vi "Meas Result Get Readings.vi"(5 "table ref":refnum<vi>, 6 "equ cct":T1, 7 "formats":T3={"mjr fmt"=enum."%_5p", "mnr fmt"=enum."%_5p", "iref fmt"=enum."%_5p", "udut fmt"=enum."%_5p", "udvm fmt"=enum."%_5p"}, 8 "error in (no error)":errorcluster, 9 "ring spot":refnum<vi>, 10 "ring phase":refnum<vi>, 11 "result":T6) -> (0 "error out":errorcluster, 1 "sweep spot index":u16, 2 "phase index":u16, 3 "readings":T4, 4 "quantities":T5)   [LabVIEW 2020]
doc: "Gets readings for selected sweep spot."
uses:
  Meas Results.ctl
  bridge/Bridge Frequency Readings Data.ctl
  drivers/TWM client/Meas Proc QWTB Spectrum Data.ctl
  drivers/TWM client/TWM Phase Info.ctl
  Meas Quantity Names.ctl
  Meas Result Formats.ctl
  Meas Result Major Format.ctl
  Impedance Equivalent Circuit.ctl
panel:
  in  "fmt":T2=enum."%_5p" caption="format"
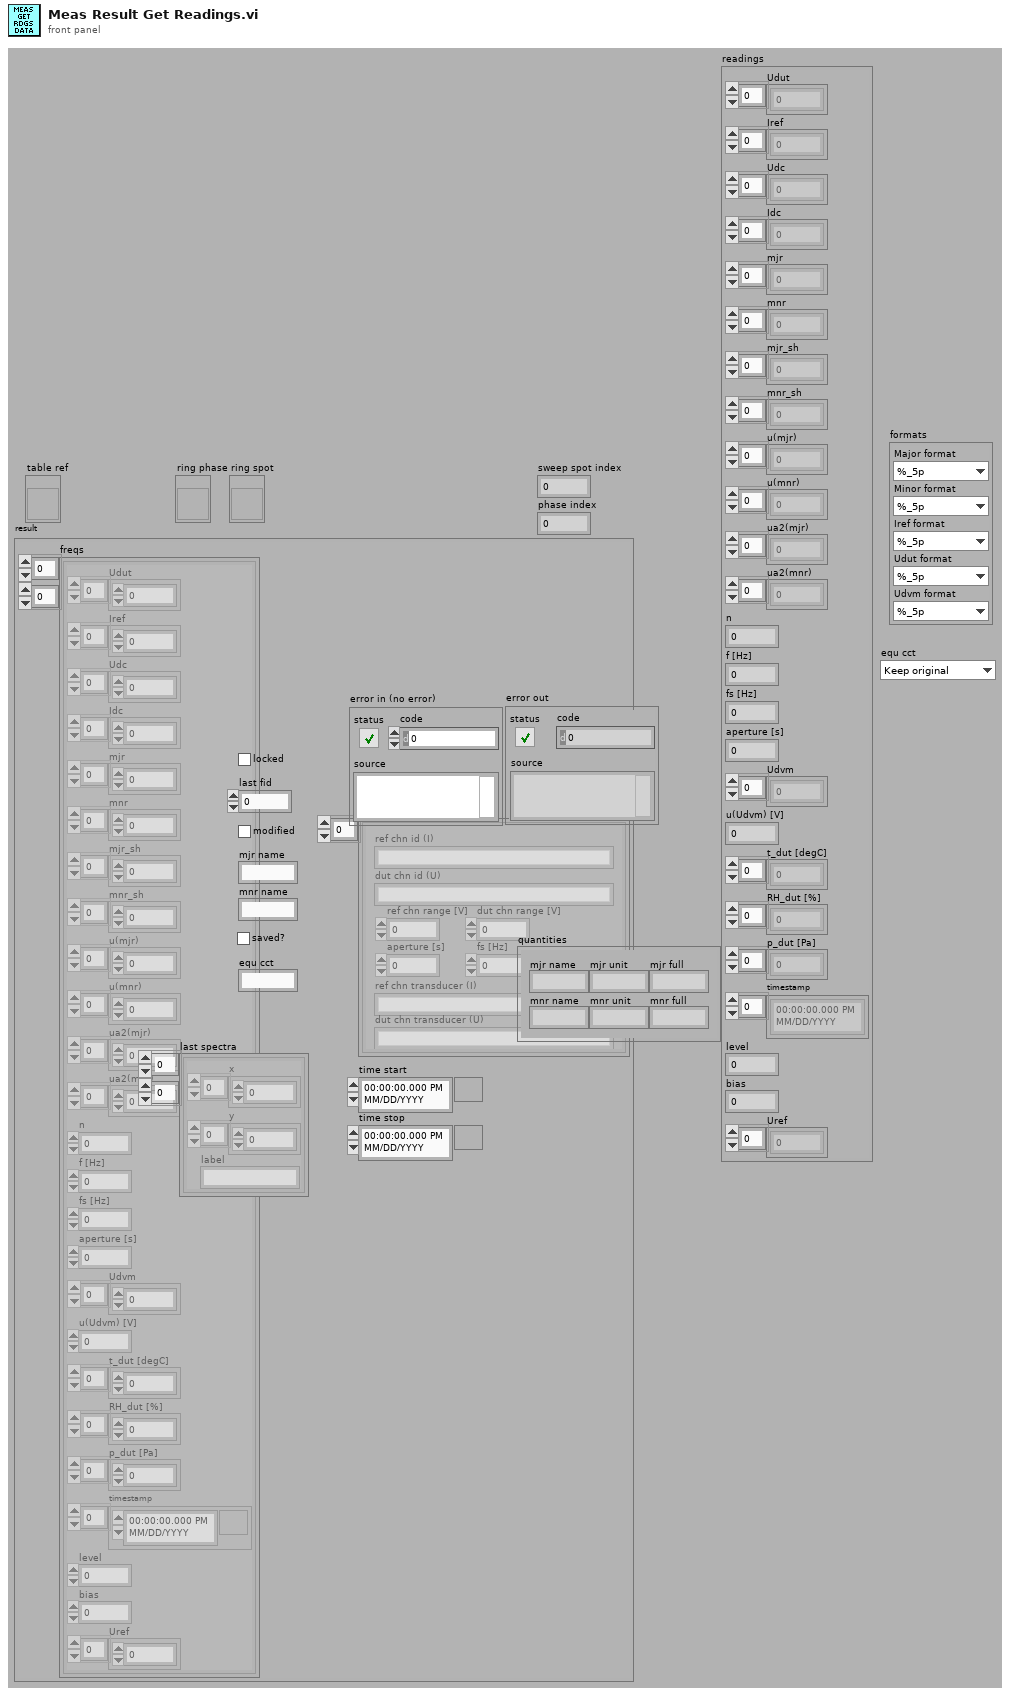
[diagram p1: front panel]
types:
  T1 = typedef "Impedance Equivalent Circuit.ctl" = enum16{"Keep original", "Rs-Xs", "Gp-Bp", "Z-phid", "Z-phir", "Y-phid", "Y-phir", "Cp-D", "Cp-Q", "Cp-Rp", "Cp-Gp", "Cs-D", "Cs-Q", "Cs-Rs", "Ls-Rs", "Ls-Q", "Rs-Tau"}
  T2 = typedef "Meas Result Major Format.ctl" = enum16{"%_3p", "%_4p", "%_5p", "%_6p", "%_7p", "%_8p", "%_5f", "%_6f", "%_7f", "%_8f", "%_5e", "%_6e", "%_7e", "%_8e", "%.4f", "%.5f", "%.6f", "%.7f"}
  T3 = typedef "Meas Result Formats.ctl" = cluster{"mjr fmt":T2, "mnr fmt":T2, "iref fmt":T2, "udut fmt":T2, "udvm fmt":T2}
  T4 = typedef "Bridge Frequency Readings Data.ctl" = cluster{"Udut":dbl[], "Iref":dbl[], "Udc":dbl[], "Idc":dbl[], "mjr":dbl[], "mnr":dbl[], "mjr_sh":dbl[], "mnr_sh":dbl[], "u(mjr)":dbl[], "u(mnr)":dbl[], "ua2(mjr)":dbl[], "ua2(mnr)":dbl[], "n":i32, "f [Hz]":dbl, "fs [Hz]":dbl, "aperture [s]":dbl, "Udvm":dbl[], "u(Udvm) [V]":dbl, "t_dut [degC]":dbl[], "RH_dut [%]":dbl[], "p_dut [Pa]":dbl[], "timestamp":timestamp[], "level":dbl, "bias":dbl, "Uref":dbl[]}
  T5 = typedef "Meas Quantity Names.ctl" = cluster{"mjr name":string, "mnr name":string, "mjr unit":string, "mnr unit":string, "mjr full":string, "mnr full":string}
  T6 = typedef "Meas Results.ctl" = cluster{"freqs":T4[][], "locked":bool, "last fid":i32, "modified":bool, "mjr name":string, "mnr name":string, "last spectra":T7[][], "saved?":bool, "TWM phase":T8[], "time start":timestamp, "time stop":timestamp, "equ cct":string}
  T7 = typedef "Meas Proc QWTB Spectrum Data.ctl" = cluster{"x":sgl[], "y":sgl[], "label":string}
  T8 = typedef "TWM Phase Info.ctl" = cluster{"ref chn id (I)":string, "dut chn id (U)":string, "ref chn range [V]":dbl, "dut chn range [V]":dbl, "aperture [s]":dbl, "fs [Hz]":dbl, "ref chn transducer (I)":string, "dut chn transducer (U)":string}
  T9 = typedef "Impedance Equivalent Circuit Type Info.ctl" = cluster{"major":string, "major unit":string, "minor":string, "minor unit":string, "combined":string, "major+unit":string, "minor+unit":string}
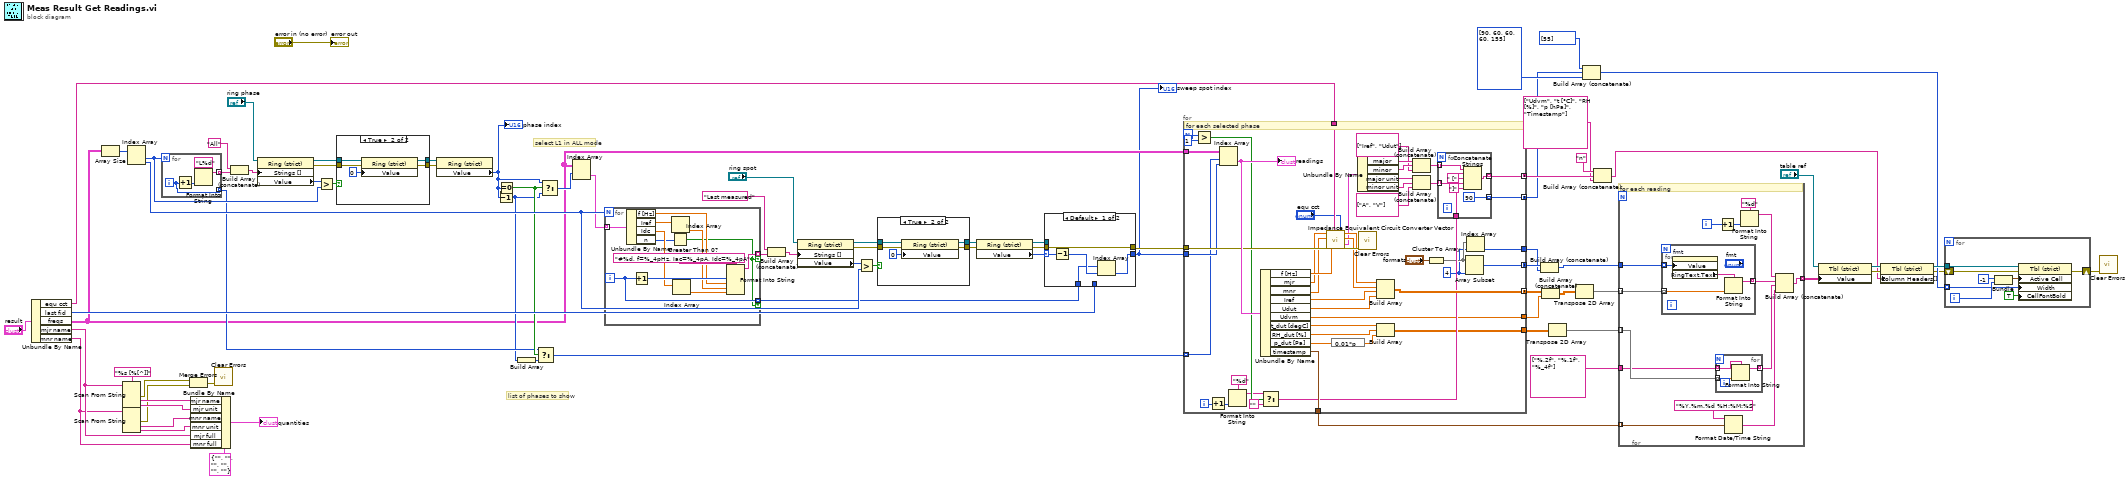
[diagram p0: block diagram]
diagram:
  w76 = "%s [%[^]]" ("format string")
  # "list of phases to show"
  # "select L1 in ALL mode"
  n1 = Unbundle By Name("result") -> ("equ cct"=w37:string, "last fid"=w41:i32, "freqs"=w24:T4[][], "mjr name"=w73:string, "mnr name"=w72:string)
  n2 = Array Size(array=w24) -> (size(s)=w67:i32[])
  n3 = Scan From String(format string=w76, input string=w73) -> (error out=w69:errorcluster, output 1=w78:string, output 2=w77:string)  [unwired: 4 in, 2 out]
  n4 = Scan From String(format string=w76, input string=w72) -> (error out=w70:errorcluster, output 1=w75:string, output 2=w74:string)  [unwired: 4 in, 2 out]
  n5 = Index Array(array=w67) -> (element #1=w64:i32, element #2=w56:i32)  [unwired: 2 in]
  n6 = for {
    N: w64 -> [_]
    tunnel: [w82] -> w33 mode=indexing
    tunnel: [w81] -> w27 mode=indexing
    i -> [w81]
    n7 = Increment(x=w81) -> (x+1=w83:i32)
    n8 = Format Into String(format string="L%d", w83) -> (resulting string=w82:string)  [unwired: 2 in, 1 out]
  }
  n9 = Merge Errors(w69, w70) -> (w68:errorcluster)
  n10 = Bundle By Name(cluster=T5 {"mjr name"="", "mnr name"="", "mjr unit"="", "mnr unit"="", "mjr full"="", "mnr full"=""} ("quantities"), "mjr name"=w78, "mjr unit"=w77, "mnr name"=w75, "mnr unit"=w74, "mjr full"=w73, "mnr full"=w72) -> (→"quantities":T5)
  n11 = call <vilib>:"Clear Errors.vi"("error in (no error)"=w68) -> ()  [unwired: 5 in, 2 out]
  n12 = Build Array (concatenate)("All", w33) -> (w32:string[])
  n13 = property class="Ring (strict)"(reference="ring phase", "Strings []"=w32) -> (reference out=w62:refnum<vi>, error out=w60:errorcluster, "Value"=w65:u16)  [unwired: 1 in]
  n14 = Greater?(x=w65, y=w64) -> (0:w63:bool)
  n15 = case shown="True" w63 {
    tunnel: w62 -> [w86 w91]
    tunnel: [w86 w89] -> w61
    tunnel: [w85 w87] -> w59
    tunnel: w60 -> [w85 w88]
    frame False {
    }
    frame True {
      n16 = property class="Ring (strict)"(reference=w91, error in=w88, "Value"=u16 0) -> (reference out=w89:refnum<vi>, error out=w87:errorcluster)
    }
  }
  n17 = property class="Ring (strict)"(reference=w61, error in=w59) -> ("Value"=w30:u16)  [unwired: 2 out]
  "phase index" <- w30
  n18 = Decrement(x=w30) -> (x-1=w25:u16)
  n19 = Equal To 0?(x=w30) -> (x = 0?=w28:bool)
  n20 = Build Array(w25) -> (w26:u16[])
  n21 = Select(t=w27, s=w28, f=w26) -> (s? t:f=w22:i32[])
  n22 = Select(t=w30, s=w28, f=w25) -> (s? t:f=w29:u16)
  n23 = Index Array(array=w24, index (row)=w29) -> (element=w48:T4[])  [unwired: 1 in]
  n24 = for {
    N: w56 -> [_]
    tunnel: [w101] -> w46 mode=indexing if=w92
    tunnel: w48 -> [w100] mode=indexing
    tunnel: [w93] -> w40 mode=indexing if=w92
    i -> [w93]
    n25 = Unbundle By Name(w100) -> ("f [Hz]"=w99:dbl, "Iref"=w98:dbl[], "Idc"=w96:dbl[], "n"=w94:i32)
    n26 = Increment(x=w93) -> (x+1=w102:i32)
    n27 = Index Array(array=w98) -> (element=w97:dbl)  [unwired: 1 in]
    n28 = Greater Than 0?(x=w94) -> (x > 0?=w92:bool)
    n29 = Index Array(array=w96) -> (element=w95:dbl)  [unwired: 1 in]
    n30 = Format Into String(format string="#%d, f=%_4pHz, Iac=%_4pA, Idc=%_4pA", w102, w99, w97, w95) -> (resulting string=w101:string)  [unwired: 2 in, 1 out]
  }
  n31 = Build Array (concatenate)("Last measured", w46) -> (w45:string[])
  n32 = property class="Ring (strict)"(reference="ring spot", "Strings []"=w45) -> (reference out=w54:refnum<vi>, error out=w55:errorcluster, "Value"=w57:u16)  [unwired: 1 in]
  n33 = Greater?(x=w57, y=w56) -> (0:w53:bool)
  n34 = case shown="True" w53 {
    tunnel: w54 -> [w105 w110]
    tunnel: [w105 w108] -> w51
    tunnel: [w104 w106] -> w52
    tunnel: w55 -> [w104 w107]
    frame False {
    }
    frame True {
      n35 = property class="Ring (strict)"(reference=w110, error in=w107, "Value"=u16 0) -> (reference out=w108:refnum<vi>, error out=w106:errorcluster)
    }
  }
  n36 = property class="Ring (strict)"(reference=w51, error in=w52) -> (reference out=w49:refnum<vi>, error out=w50:errorcluster, "Value"=w42:u16)
  n37 = case shown="Default" w42 {
    selector: w42 -> [w115 _]
    tunnel: w50 -> [w114 w116]
    tunnel: w49 -> [_ _]
    tunnel: [w112 w117] -> w23
    tunnel: w41 -> [_ w117]
    tunnel: [w114 w116] -> w38
    tunnel: w40 -> [w111 _]
    frame Default {
      n38 = Decrement(x=w115) -> (x-1=w113:u16)
      n39 = Index Array(array=w111, index=w113) -> (element=w112:i32)
    }
    frame 0 {
    }
  }
  "sweep spot index" <- w23
  n40 = for {
    N -> [w139]
    tunnel: [w144] -> w13 mode=concatenating
    tunnel: [w124] -> w15 mode=concatenating
    tunnel: w38 -> [w157]
    tunnel: w37 -> [w153]
    tunnel: [w149] -> w34
    tunnel: w24 -> [w147]
    tunnel: w23 -> [w146]
    tunnel: w22 -> [w145] mode=indexing
    tunnel: [w125] -> w18 mode=concatenating
    tunnel: [w121] -> w14
    tunnel: [w120] -> w12
    tunnel: [w119] -> w20
    tunnel: [w118] -> w5 mode=concatenating
    i -> [w142]
    w122 = 4 ("length")
    # "for each selected phase"
    n41 = Greater?(x=w139, y=1) -> (0:w137:bool)
    n42 = Increment(x=w142) -> (x+1=w141:i32)
    n43 = Index Array(array=w147, index (row)=w145, index (col)=w146) -> (element=w165:T4)
    "readings" <- w165
    n44 = Format Into String(format string="%d", w141) -> (resulting string=w136:string)  [unwired: 2 in, 1 out]
    n45 = Unbundle By Name(w165) -> ("f [Hz]"=w156:dbl, "mjr"=w155:dbl[], "mnr"=w154:dbl[], "Iref"=w164:dbl[], "Udut"=w163:dbl[], "Udvm"=w120:dbl[], "t_dut [degC]"=w161:dbl[], "RH_dut [%]"=w160:dbl[], "p_dut [Pa]"=w159:dbl[], "timestamp"=w149:timestamp[])
    n46 = Select(t=w136, s=w137, f="") -> (s? t:f=w134:string)
    n47 = call "Impedance Equivalent Circuit Converter Vector.vi"("major in"=w155, "minor in"=w154, "error in (no error)"=w157, "f scalar [Hz]"=w156, "type in by string"=w153, "type out"="equ cct") -> ("major out"=w151:dbl[], "minor out"=w150:dbl[], "type out info"=w143:T9, "error out"=w158:errorcluster)  [unwired: 8 in, 2 out]
    n48 = expression code="0.01*p"(w159) -> (w148:dbl[])
    n49 = Unbundle By Name(w143) -> ("major"=w133:string, "minor"=w132:string, "major unit"=w130:string, "minor unit"=w129:string)
    n50 = call <vilib>:"Clear Errors.vi"("error in (no error)"=w158) -> ()  [unwired: 5 in, 2 out]
    n51 = Build Array(w151, w150, w164, w163) -> (w144:dbl[][])
    n52 = Build Array(w161, w160, w148) -> (w119:dbl[][])
    n53 = Build Array (concatenate)(w133, w132, string[] ["Iref", "Udut"] ("element")) -> (w127:string[])
    n54 = Build Array (concatenate)(w130, w129, string[] ["A", "V"] ("element")) -> (w126:string[])
    n55 = Cluster To Array(cluster="formats") -> (array=w123:T2[])
    n56 = for {
      tunnel: w134 -> [w172]
      tunnel: w127 -> [w170] mode=indexing
      tunnel: w126 -> [w169] mode=indexing
      tunnel: [w168] -> w125 mode=indexing
      tunnel: [u32 90 ("Width")] -> w118 mode=indexing
      n57 = Concatenate Strings(w170, w172, " [" ("string"), w169, "]" ("string")) -> (w168:string)
    }
    n58 = Array Subset(array=w123, length=w122) -> (w124:T2[])  [unwired: 1 in]
    n59 = Index Array(array=w123, index=w122) -> (element=w121:T2)
  }
  n60 = Build Array (concatenate)(w15, w14) -> (w9:T2[])
  n61 = Build Array (concatenate)(w13, w12) -> (w11:dbl[][])
  n62 = Transpose 2D Array(2D array=w20) -> (transposed array=w19:dbl[][])
  n63 = Transpose 2D Array(2D array=w11) -> (transposed array=w21:dbl[][])
  n64 = Build Array (concatenate)(u32[] [55] ("Array"), w5, u32[] [90, 60, 60, 60, 155] ("Array")) -> (w3:u32[])
  n65 = Build Array (concatenate)("n" ("element"), w18, string[] ["Udvm", "t [°C]", "RH [%]", "p [hPa]", "Timestamp"] ("element")) -> (w10:string[])
  n66 = for {
    tunnel: w21 -> [w183] mode=indexing
    tunnel: [w180] -> w47 mode=indexing
    tunnel: w9 -> [w179]
    tunnel: w19 -> [w178] mode=indexing
    tunnel: string[] ["%.2f", "%.1f", "%_4f"] -> [w177]
    tunnel: w34 -> [w174] mode=indexing
    i -> [w186]
    # "for each reading"
    n67 = for {
      tunnel: w183 -> [w193] mode=indexing
      tunnel: [w192] -> w182 mode=indexing
      tunnel: w179 -> [w191] mode=indexing
      n68 = property on="fmt" class="Enum (strict)"("Value"=w191) -> ("RingText.Text"=w190:string)  [unwired: 2 in, 2 out]
      n69 = Format Into String(format string=w190, w193) -> (resulting string=w192:string)  [unwired: 2 in, 1 out]
    }
    n70 = for {
      tunnel: w178 -> [w189] mode=indexing
      tunnel: [w188] -> w176 mode=indexing
      tunnel: w177 -> [w187] mode=indexing
      n71 = Format Into String(format string=w187, w189) -> (resulting string=w188:string)  [unwired: 2 in, 1 out]
    }
    n72 = Increment(x=w186) -> (x+1=w184:i32)
    n73 = Format Date/Time String(time format string (%c)="%Y.%m.%d %H:%M:%S" ("format string"), seconds (now)=w174) -> (date/time string=w173:string)  [unwired: 1 in]
    n74 = Format Into String(format string="%d", w184) -> (resulting string=w181:string)  [unwired: 2 in, 1 out]
    n75 = Build Array (concatenate)(w181, w182, w176, w173) -> (w180:string[])
  }
  n76 = property class="Tbl (strict)"(reference="table ref", "Value"=w47) -> (reference out=w35:refnum<vi>, error out=w36:errorcluster)  [unwired: 1 in]
  n77 = property class="Tbl (strict)"(reference=w35, error in=w36, "Column Headers[]"=w10) -> (reference out=w4:refnum<vi>, error out=w2:errorcluster)
  n78 = for {
    tunnel: w4 -> [w201]
    tunnel: w3 -> [w197] mode=indexing
    shift-right: [w194] -> w1
    shift-left: w2 -> [w195]
    i -> [w199]
    n79 = Bundle(-1, w199) -> (w200:cluster{i32, i32})  [unwired: 1 in]
    n80 = property class="Tbl (strict)"(reference=w201, error in=w195, "Active Cell"=w200, "Width"=w197, "CellFontBold"=TRUE ("Active Cell:Cell Font:Bold")) -> (error out=w194:errorcluster)  [unwired: 1 out]
  }
  n81 = call <vilib>:"Clear Errors.vi"("error in (no error)"=w1) -> ()  [unwired: 5 in, 2 out]
  "error out" <- "error in (no error)"
